vi "Signal 2 String.vi"(1 "Signal":dbl[](array[numeric]) format="%.2f") -> (0 "String":string)   [LabVIEW 2010]
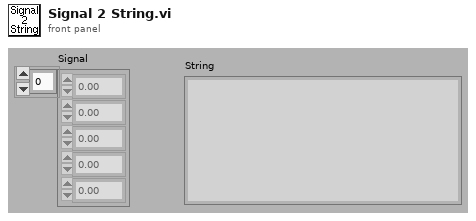
[diagram p1: front panel]
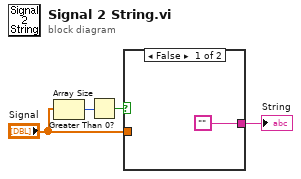
[diagram p0: block diagram]
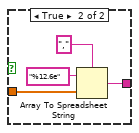
[diagram p2: hidden frame]
diagram:
  n1 = Array Size(array="Signal") -> (size(s)=w2:i32)
  n2 = Greater Than 0?(x=w2) -> (x > 0?=w3:bool)
  n3 = case shown="False" w3 {
    tunnel: "Signal" -> [_ w9]
    tunnel: ["" w6] -> w4
    frame False {
    }
    frame True {
      n4 = Array To Spreadsheet String(delimiter (Tab)=",", array=w9, 3:"%12.6e" ("format string")) -> (spreadsheet string=w6:string)
    }
  }
  "String" <- w4
